vi "Finalize Shared Resources.vi"(8 "error in":errorcluster, 11 "RTStateVariables in":T1 {"Inline Execution Units"."Outgoing Data References"."Data Reference" format="%.0x"; "Inline Execution Units"."Incoming Data References" format="%.0x"}) -> (0 "error out":errorcluster, 3 "RTStateVariables out":T1 {"Inline Execution Units"."Outgoing Data References"."Data Reference" format="%.0x"; "Inline Execution Units"."Incoming Data References" format="%.0x"})   [LabVIEW 2020, in "AIM MIL-STD-1553 Engine.lvlib" / "Custom Device.lvlib"]
uses:
  Custom Device.lvlib
  Interfaces/Shared Resources/Shared Resources.lvclass
  <vilib>/NI/NIVS Inline Async API/_VS Inline Async API/VS Inline Async API/VS Inline Async API.lvclass
  RTStateVariables.ctl
  <vilib>/NI VeriStand/Custom Device API/Data Reference.ctl
  <vilib>/NI VeriStand/Custom Device API/Custom Device API.lvlib
  <vilib>/NI VeriStand/Custom Device API/Block Data Reference.ctl
  Interfaces/Execution Unit/Execution Unit.lvclass
  Inline Execution Unit Runtime Information.ctl
  Asynchronous Execution Unit Runtime Information.ctl
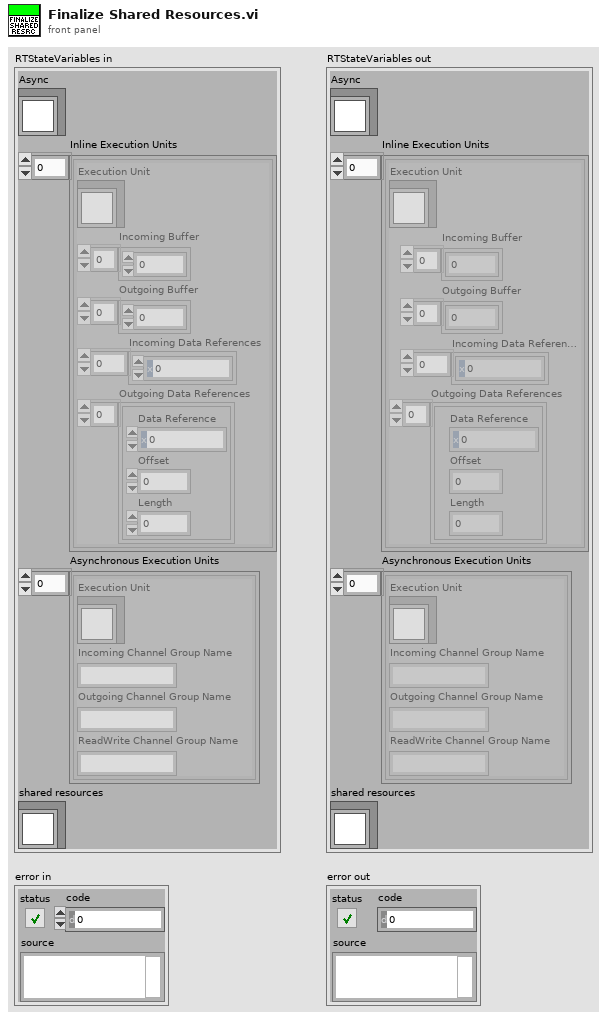
[diagram p1: front panel]
types:
  T1 = typedef "AIM MIL-STD-1553 Engine.lvlib/Custom Device.lvlib/RTStateVariables.ctl" = cluster{"Async":refnum<class "VS Inline Async API.lvclass">, "Inline Execution Units":T2[], "Asynchronous Execution Units":T5[], "shared resources":refnum<class "Shared Resources.lvclass">}
  T2 = typedef "AIM MIL-STD-1553 Engine.lvlib/Custom Device.lvlib/Inline Execution Unit Runtime Information.ctl" = cluster{"Execution Unit":refnum<class "Execution Unit.lvclass">, "Incoming Buffer":dbl[], "Outgoing Buffer":dbl[], "Incoming Data References":T3[], "Outgoing Data References":T4[]}
  T3 = typedef "Custom Device API.lvlib/Data Reference.ctl" = i32
  T4 = typedef "Custom Device API.lvlib/Block Data Reference.ctl" = cluster{"Data Reference":T3, "Offset":u64, "Length":u64}
  T5 = typedef "AIM MIL-STD-1553 Engine.lvlib/Custom Device.lvlib/Asynchronous Execution Unit Runtime Information.ctl" = cluster{"Execution Unit":refnum<class "Execution Unit.lvclass">, "Incoming Channel Group Name":string, "Outgoing Channel Group Name":string, "ReadWrite Channel Group Name":string}
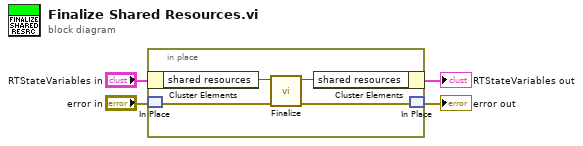
[diagram p0: block diagram]
diagram:
  n1 = in-place {
    n2 = in-place-cluster #1("RTStateVariables in") -> ("shared resources"=w5:refnum<class "Shared Resources.lvclass">)
    n3 = in-place-match #2("error in") -> (w8:errorcluster)
    n4 = call-dynamic "Finalize.vi"("error in"=w8, "shared resources in"=w5) -> ("error out"=w7:errorcluster, "shared resources out"=w6:refnum<class "Shared Resources.lvclass">)  [unwired: 8 in]
    n5 = in-place-cluster #1("shared resources"=w6) -> (→"RTStateVariables out":T1)
    n6 = in-place-match #2(w7) -> (→"error out":errorcluster)
  }
